vi "FGV GAGE Zero.vi"(7 "CMD":T1, 8 "error in (no error)":errorcluster, 9 "index":i32, 11 "input":dbl) -> (0 "error out":errorcluster, 3 "output":dbl[](array[numeric]))   [LabVIEW 2020]
uses:
  PCT FGV CMD.ctl
panel:
  # "0 - Gage at Zero\n1 - GF"
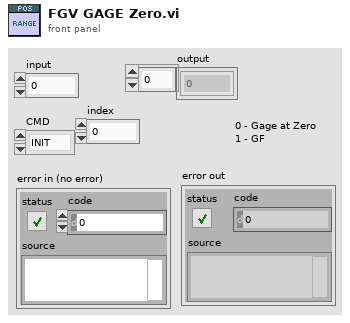
[diagram p1: front panel]
types:
  T1 = typedef "PCT FGV CMD.ctl" = enum16{"INIT", "GET", "SET"}
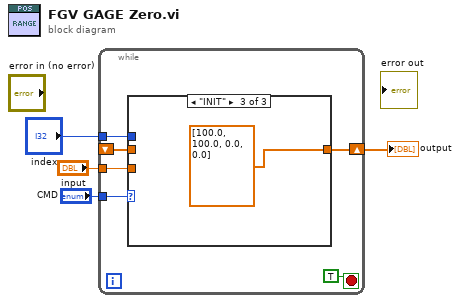
[diagram p0: block diagram]
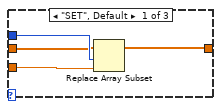
[diagram p2: hidden frame]
diagram:
  n1 = while {
    tunnel: "input" -> [w8]
    tunnel: "CMD" -> [w10]
    shift-right: [w7] -> w4
    shift-left: _ -> [w9]
    tunnel: "index" -> [w5]
    stop <- TRUE stop-if-true
    n2 = case shown="\"INIT\"" w10 {
      tunnel: w9 -> [w12 w15 _]
      tunnel: w8 -> [w11 _ _]
      tunnel: [w14 w15 dbl[] [100.0, 100.0, 0.0, 0.0] ("input")] -> w7
      tunnel: w5 -> [w13 _ _]
      frame "SET", Default {
        n3 = Replace Array Subset(array=w12, new element=w11, index=w13) -> (w14:dbl[])
      }
      frame "GET" {
      }
      frame "INIT" {
      }
    }
  }
  "output" <- w4
